vi "Polar to Cartesian (subVI - Hideyoshi ver).vi"(9 "Angle (rads)":dbl, 10 "Magnitude (r)":dbl) -> (1 "y (r*sin(theta))":dbl, 2 "x (r*cos(theta))":dbl)   [LabVIEW 2016]
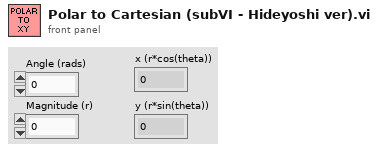
[diagram p1: front panel]
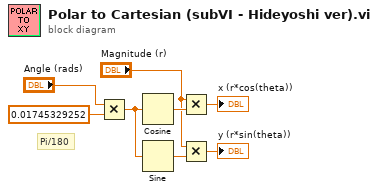
[diagram p0: block diagram]
diagram:
  # "Pi/180"
  n1 = Multiply(x="Angle (rads)", y=0.01745329252 ("x")) -> (x*y=w6:dbl)
  n2 = Cosine(x=w6) -> (cos(x)=w3:dbl)
  n3 = Sine(x=w6) -> (sin(x)=w2:dbl)
  n4 = Multiply(x="Magnitude (r)", y=w3) -> (x*y=→"x (r*cos(theta))":dbl)
  n5 = Multiply(x="Magnitude (r)", y=w2) -> (x*y=→"y (r*sin(theta))":dbl)
